vi "Begin.vi"(8 "error in":errorcluster) -> (0 "error out":errorcluster)   [LabVIEW 2018]
doc: "Called before other user functions, this VI is expected to open initial I/O refnums, load in file data, and do all program initialization. Notice that the <B>error out</B> terminal is simply used for data flow. Wiring it to other structures or subVIs ensures that this VI runs first."
uses:
  Robot Global Data.vi
  <vilib>/Rock Robotics/WPI/DriverStation/WPI_DriverStationRobotMode2.ctl
  <vilib>/Rock Robotics/WPI/Counter/WPI_CounterDigitalInputToDigitalSource.vi
  <vilib>/Rock Robotics/SystemInterfaces/DIO/FPGA_DIOChannel.ctl
  <vilib>/Rock Robotics/WPI/Solenoid/WPI_SolenoidOpenDouble.vi
  <vilib>/Rock Robotics/WPI/Solenoid/WPI_SolenoidSetEnum.vi
  <vilib>/Rock Robotics/WPI/Solenoid/WPI_SolenoidChannel.ctl
  <vilib>/Rock Robotics/SystemInterfaces/spilib/spi_bus.ctl
  <vilib>/Rock Robotics/WPI/Joystick/WPI_JoystickDeviceEnum.ctl
  <vilib>/Rock Robotics/SystemInterfaces/AI/FPGA_AIChannel.ctl
  <vilib>/Rock Robotics/WPI/Gyro/WPI_GyroXRS450_SPI_Open.vi
  <vilib>/Rock Robotics/WPI/Switch/WPI_SwitchOpenLimit.vi
  <vilib>/Rock Robotics/SystemInterfaces/DIO/FPGA_DIOPWMChannel.ctl
  <vilib>/Rock Robotics/WPI/PWM/WPI_PWMDeadband.ctl
  <vilib>/Rock Robotics/WPI/MotorControl/WPI_MotorControlType.ctl
  <vilib>/Rock Robotics/WPI/MotorControl/WPI_MotorControlDeviceRef.ctl
  <vilib>/Rock Robotics/WPI/RobotDrive/WPI_RobotDriveDevRef.ctl
  TeleopAutoCluster.ctl
  <vilib>/Rock Robotics/WPI/Joystick/WPI_JoystickDevRef.ctl
  <vilib>/Rock Robotics/WPI/Encoder/WPI_EncoderDevRef.ctl
  <vilib>/Rock Robotics/SystemInterfaces/Encoder/FPGA_EncoderIdx.ctl
  <vilib>/Rock Robotics/WPI/Encoder/WPI_EncoderType.ctl
  <vilib>/Rock Robotics/SystemInterfaces/Counter/FPGA_CounterCtrSystemIndex.ctl
  <vilib>/Rock Robotics/WPI/Gyro/WPI_GyroDevRef.ctl
  PTCluster.ctl
  <vilib>/Rock Robotics/WPI/Solenoid/WPI_SolenoidDevRef.ctl
  <vilib>/Rock Robotics/WPI/Switch/WPI_SwitchDevRef.ctl
  <vilib>/Rock Robotics/WPI/Potentiometer/WPI_PotentiometerDevRef.ctl
panel:
  out "PT Cluster Out":T1={"Elevator Encoder"={"DevStatus"={"status"=FALSE, "code"=0, "source"=""}, "EncoderIndex"=enum."Invalid", "CounterIndex"=enum."Ctr 1", "DistancePerCount"=2.0, "Decoding Type"=enum."4x"}, "Solenoid0"={"DevStatus"={"status"=FALSE, "code"=0, "source"=""}, "Pneumatics Control Module"=0, "Forward Solenoid Channel"=enum."Invalid", "Reverse Solenoid Channel"=enum."Invalid"}, "Solenoid1"={"DevStatus"={"status"=FALSE, "code"=0, "source"=""}, "Pneumatics Control Module"=0, "Forward Solenoid Channel"=enum."Invalid", "Reverse Solenoid Channel"=enum."Invalid"}, "Solenoid2"={"DevStatus"={"status"=FALSE, "code"=0, "source"=""}, "Pneumatics Control Module"=0, "Forward Solenoid Channel"=enum."Invalid", "Reverse Solenoid Channel"=enum."Invalid"}, "Solenoid3"={"DevStatus"={"status"=FALSE, "code"=0, "source"=""}, "Pneumatics Control Module"=0, "Forward Solenoid Channel"=enum."Invalid", "Reverse Solenoid Channel"=enum."Invalid"}, "Solenoid4"={"DevStatus"={"status"=FALSE, "code"=0, "source"=""}, "Pneumatics Control Module"=0, "Forward Solenoid Channel"=enum."Invalid", "Reverse Solenoid Channel"=enum."Invalid"}, "Elevator Master"={"DeviceStatus"={"status"=FALSE, "code"=0, "source"=""}, "Type"=enum."PWM", "PWM"={"PWM Channel"=enum."Invalid", "DeadBand"={"Name"="", "maxPositivePwm"=0, "minPositivePwm"=0, "centerPwm"=0, "maxNegativePwm"=0, "minNegativePwm"=0, "angularRange"=0}}, "CAN"={"Device Number"=0, "SetOutput VI Ref"=variant(refnum<vi> refnum), "GetOutput VI Ref"=variant(refnum<vi> refnum), "Enable VI Ref"=variant(refnum<vi> refnum), "Disable VI Ref"=variant(refnum<vi> refnum), "Data"=variant}, "Invert"=FALSE, "DIO PWM"={"PWM \"Enable\" Channel"=enum."Invalid", "DIOChannel"=enum."Invalid", "PWM Rate"=0.0}}, "Elevator Master 2"={"DeviceStatus"={"status"=FALSE, "code"=0, "source"=""}, "Type"=enum."PWM", "PWM"={"PWM Channel"=enum."Invalid", "DeadBand"={"Name"="", "maxPositivePwm"=0, "minPositivePwm"=0, "centerPwm"=0, "maxNegativePwm"=0, "minNegativePwm"=0, "angularRange"=0}}, "CAN"={"Device Number"=0, "SetOutput VI Ref"=variant(refnum<vi> refnum), "GetOutput VI Ref"=variant(refnum<vi> refnum), "Enable VI Ref"=variant(refnum<vi> refnum), "Disable VI Ref"=variant(refnum<vi> refnum), "Data"=variant}, "Invert"=FALSE, "DIO PWM"={"PWM \"Enable\" Channel"=enum."Invalid", "DIOChannel"=enum."Invalid", "PWM Rate"=0.0}}, "Elevator Master 3"={"DeviceStatus"={"status"=FALSE, "code"=0, "source"=""}, "Type"=enum."PWM", "PWM"={"PWM Channel"=enum."Invalid", "DeadBand"={"Name"="", "maxPositivePwm"=0, "minPositivePwm"=0, "centerPwm"=0, "maxNegativePwm"=0, "minNegativePwm"=0, "angularRange"=0}}, "CAN"={"Device Number"=0, "SetOutput VI Ref"=variant(refnum<vi> refnum), "GetOutput VI Ref"=variant(refnum<vi> refnum), "Enable VI Ref"=variant(refnum<vi> refnum), "Disable VI Ref"=variant(refnum<vi> refnum), "Data"=variant}, "Invert"=FALSE, "DIO PWM"={"PWM \"Enable\" Channel"=enum."Invalid", "DIOChannel"=enum."Invalid", "PWM Rate"=0.0}}, "Elevator Master 4"={"DeviceStatus"={"status"=FALSE, "code"=0, "source"=""}, "Type"=enum."PWM", "PWM"={"PWM Channel"=enum."Invalid", "DeadBand"={"Name"="", "maxPositivePwm"=0, "minPositivePwm"=0, "centerPwm"=0, "maxNegativePwm"=0, "minNegativePwm"=0, "angularRange"=0}}, "CAN"={"Device Number"=0, "SetOutput VI Ref"=variant(refnum<vi> refnum), "GetOutput VI Ref"=variant(refnum<vi> refnum), "Enable VI Ref"=variant(refnum<vi> refnum), "Disable VI Ref"=variant(refnum<vi> refnum), "Data"=variant}, "Invert"=FALSE, "DIO PWM"={"PWM \"Enable\" Channel"=enum."Invalid", "DIOChannel"=enum."Invalid", "PWM Rate"=0.0}}, "Elevator Bottom Out"={"DevStatus"={"status"=FALSE, "code"=0, "source"=""}, "DIO Channel"=enum."Invalid", "CntIndex"=enum."Invalid", "Normally Closed"=FALSE}, "Pot Moto"={"DevStatus"={"status"=FALSE, "code"=0, "source"=""}, "Analog Channel"=enum."Invalid", "Invert Output"=FALSE}, "Pot  Arm"={"DevStatus"={"status"=FALSE, "code"=0, "source"=""}, "Analog Channel"=enum."Invalid", "Invert Output"=FALSE}, "Elevator Master 5"={"DeviceStatus"={"status"=FALSE, "code"=0, "source"=""}, "Type"=enum."PWM", "PWM"={"PWM Channel"=enum."Invalid", "DeadBand"={"Name"="", "maxPositivePwm"=0, "minPositivePwm"=0, "centerPwm"=0, "maxNegativePwm"=0, "minNegativePwm"=0, "angularRange"=0}}, "CAN"={"Device Number"=0, "SetOutput VI Ref"=variant(refnum<vi> refnum), "GetOutput VI Ref"=variant(refnum<vi> refnum), "Enable VI Ref"=variant(refnum<vi> refnum), "Disable VI Ref"=variant(refnum<vi> refnum), "Data"=variant}, "Invert"=FALSE, "DIO PWM"={"PWM \"Enable\" Channel"=enum."Invalid", "DIOChannel"=enum."Invalid", "PWM Rate"=0.0}}, "Hatch Detection"={"DevStatus"={"status"=FALSE, "code"=0, "source"=""}, "DIO Channel"=enum."Invalid", "CntIndex"=enum."Invalid", "Normally Closed"=FALSE}, "Infrared"={"DevStatus"={"status"=FALSE, "code"=0, "source"=""}, "DIO Channel"=enum."Invalid", "CntIndex"=enum."Invalid", "Normally Closed"=FALSE}}
  in  "PT Cluster":T1={"Elevator Encoder"={"DevStatus"={"status"=FALSE, "code"=0, "source"=""}, "EncoderIndex"=enum."Invalid", "CounterIndex"=enum."Ctr 1", "DistancePerCount"=2.0, "Decoding Type"=enum."4x"}, "Solenoid0"={"DevStatus"={"status"=FALSE, "code"=0, "source"=""}, "Pneumatics Control Module"=0, "Forward Solenoid Channel"=enum."Invalid", "Reverse Solenoid Channel"=enum."Invalid"}, "Solenoid1"={"DevStatus"={"status"=FALSE, "code"=0, "source"=""}, "Pneumatics Control Module"=0, "Forward Solenoid Channel"=enum."Invalid", "Reverse Solenoid Channel"=enum."Invalid"}, "Solenoid2"={"DevStatus"={"status"=FALSE, "code"=0, "source"=""}, "Pneumatics Control Module"=0, "Forward Solenoid Channel"=enum."Invalid", "Reverse Solenoid Channel"=enum."Invalid"}, "Solenoid3"={"DevStatus"={"status"=FALSE, "code"=0, "source"=""}, "Pneumatics Control Module"=0, "Forward Solenoid Channel"=enum."Invalid", "Reverse Solenoid Channel"=enum."Invalid"}, "Solenoid4"={"DevStatus"={"status"=FALSE, "code"=0, "source"=""}, "Pneumatics Control Module"=0, "Forward Solenoid Channel"=enum."Invalid", "Reverse Solenoid Channel"=enum."Invalid"}, "Elevator Master"={"DeviceStatus"={"status"=FALSE, "code"=0, "source"=""}, "Type"=enum."PWM", "PWM"={"PWM Channel"=enum."Invalid", "DeadBand"={"Name"="", "maxPositivePwm"=0, "minPositivePwm"=0, "centerPwm"=0, "maxNegativePwm"=0, "minNegativePwm"=0, "angularRange"=0}}, "CAN"={"Device Number"=0, "SetOutput VI Ref"=variant(refnum<vi> refnum), "GetOutput VI Ref"=variant(refnum<vi> refnum), "Enable VI Ref"=variant(refnum<vi> refnum), "Disable VI Ref"=variant(refnum<vi> refnum), "Data"=variant}, "Invert"=FALSE, "DIO PWM"={"PWM \"Enable\" Channel"=enum."Invalid", "DIOChannel"=enum."Invalid", "PWM Rate"=0.0}}, "Elevator Master 2"={"DeviceStatus"={"status"=FALSE, "code"=0, "source"=""}, "Type"=enum."PWM", "PWM"={"PWM Channel"=enum."Invalid", "DeadBand"={"Name"="", "maxPositivePwm"=0, "minPositivePwm"=0, "centerPwm"=0, "maxNegativePwm"=0, "minNegativePwm"=0, "angularRange"=0}}, "CAN"={"Device Number"=0, "SetOutput VI Ref"=variant(refnum<vi> refnum), "GetOutput VI Ref"=variant(refnum<vi> refnum), "Enable VI Ref"=variant(refnum<vi> refnum), "Disable VI Ref"=variant(refnum<vi> refnum), "Data"=variant}, "Invert"=FALSE, "DIO PWM"={"PWM \"Enable\" Channel"=enum."Invalid", "DIOChannel"=enum."Invalid", "PWM Rate"=0.0}}, "Elevator Master 3"={"DeviceStatus"={"status"=FALSE, "code"=0, "source"=""}, "Type"=enum."PWM", "PWM"={"PWM Channel"=enum."Invalid", "DeadBand"={"Name"="", "maxPositivePwm"=0, "minPositivePwm"=0, "centerPwm"=0, "maxNegativePwm"=0, "minNegativePwm"=0, "angularRange"=0}}, "CAN"={"Device Number"=0, "SetOutput VI Ref"=variant(refnum<vi> refnum), "GetOutput VI Ref"=variant(refnum<vi> refnum), "Enable VI Ref"=variant(refnum<vi> refnum), "Disable VI Ref"=variant(refnum<vi> refnum), "Data"=variant}, "Invert"=FALSE, "DIO PWM"={"PWM \"Enable\" Channel"=enum."Invalid", "DIOChannel"=enum."Invalid", "PWM Rate"=0.0}}, "Elevator Master 4"={"DeviceStatus"={"status"=FALSE, "code"=0, "source"=""}, "Type"=enum."PWM", "PWM"={"PWM Channel"=enum."Invalid", "DeadBand"={"Name"="", "maxPositivePwm"=0, "minPositivePwm"=0, "centerPwm"=0, "maxNegativePwm"=0, "minNegativePwm"=0, "angularRange"=0}}, "CAN"={"Device Number"=0, "SetOutput VI Ref"=variant(refnum<vi> refnum), "GetOutput VI Ref"=variant(refnum<vi> refnum), "Enable VI Ref"=variant(refnum<vi> refnum), "Disable VI Ref"=variant(refnum<vi> refnum), "Data"=variant}, "Invert"=FALSE, "DIO PWM"={"PWM \"Enable\" Channel"=enum."Invalid", "DIOChannel"=enum."Invalid", "PWM Rate"=0.0}}, "Elevator Bottom Out"={"DevStatus"={"status"=FALSE, "code"=0, "source"=""}, "DIO Channel"=enum."Invalid", "CntIndex"=enum."Invalid", "Normally Closed"=FALSE}, "Pot Moto"={"DevStatus"={"status"=FALSE, "code"=0, "source"=""}, "Analog Channel"=enum."Invalid", "Invert Output"=FALSE}, "Pot  Arm"={"DevStatus"={"status"=FALSE, "code"=0, "source"=""}, "Analog Channel"=enum."Invalid", "Invert Output"=FALSE}, "Elevator Master 5"={"DeviceStatus"={"status"=FALSE, "code"=0, "source"=""}, "Type"=enum."PWM", "PWM"={"PWM Channel"=enum."Invalid", "DeadBand"={"Name"="", "maxPositivePwm"=0, "minPositivePwm"=0, "centerPwm"=0, "maxNegativePwm"=0, "minNegativePwm"=0, "angularRange"=0}}, "CAN"={"Device Number"=0, "SetOutput VI Ref"=variant(refnum<vi> refnum), "GetOutput VI Ref"=variant(refnum<vi> refnum), "Enable VI Ref"=variant(refnum<vi> refnum), "Disable VI Ref"=variant(refnum<vi> refnum), "Data"=variant}, "Invert"=FALSE, "DIO PWM"={"PWM \"Enable\" Channel"=enum."Invalid", "DIOChannel"=enum."Invalid", "PWM Rate"=0.0}}, "Hatch Detection"={"DevStatus"={"status"=FALSE, "code"=0, "source"=""}, "DIO Channel"=enum."Invalid", "CntIndex"=enum."Invalid", "Normally Closed"=FALSE}, "Infrared"={"DevStatus"={"status"=FALSE, "code"=0, "source"=""}, "DIO Channel"=enum."Invalid", "CntIndex"=enum."Invalid", "Normally Closed"=FALSE}}
  out "Teleop/Auto output cluster out":T16={"X Joystick"={"Device"=enum."USB 0"}, "Y Joystick"={"Device"=enum."USB 0"}, "Controller"={"Device"=enum."USB 0"}, "Right Drive Encoder"={"DevStatus"={"status"=FALSE, "code"=0, "source"=""}, "EncoderIndex"=enum."Invalid", "CounterIndex"=enum."Ctr 1", "DistancePerCount"=2.0, "Decoding Type"=enum."4x"}, "Left Drive Encoder"={"DevStatus"={"status"=FALSE, "code"=0, "source"=""}, "EncoderIndex"=enum."Invalid", "CounterIndex"=enum."Ctr 1", "DistancePerCount"=2.0, "Decoding Type"=enum."4x"}, "Gyro"={"DevStatus"={"status"=FALSE, "code"=0, "source"=""}, "Analog Channel"=enum."AI 1", "Gain (VoltsPerDegree/Second)"=0.0, "Gyro Type"=enum."Analog", "Handle"=0, "SPI Bus"=enum."Invalid", "Device Found"=FALSE, "Sample Rate"=1.0, "Calibrate On Open"=FALSE, "Offset"=0.0}, "DriveMotors"={"DevStatus"={"status"=FALSE, "code"=0, "source"=""}, "Motors[]"=[], "Square Inputs"=FALSE, "Max Output"=1.0}} {"Gyro"."Sample Rate" min=0.25 max=100.0 step=0.25}
  in  "Teleop/Auto output cluster":T16={"X Joystick"={"Device"=enum."USB 0"}, "Y Joystick"={"Device"=enum."USB 0"}, "Controller"={"Device"=enum."USB 0"}, "Right Drive Encoder"={"DevStatus"={"status"=FALSE, "code"=0, "source"=""}, "EncoderIndex"=enum."Invalid", "CounterIndex"=enum."Ctr 1", "DistancePerCount"=2.0, "Decoding Type"=enum."4x"}, "Left Drive Encoder"={"DevStatus"={"status"=FALSE, "code"=0, "source"=""}, "EncoderIndex"=enum."Invalid", "CounterIndex"=enum."Ctr 1", "DistancePerCount"=2.0, "Decoding Type"=enum."4x"}, "Gyro"={"DevStatus"={"status"=FALSE, "code"=0, "source"=""}, "Analog Channel"=enum."AI 1", "Gain (VoltsPerDegree/Second)"=0.0, "Gyro Type"=enum."Analog", "Handle"=0, "SPI Bus"=enum."Invalid", "Device Found"=FALSE, "Sample Rate"=1.0, "Calibrate On Open"=FALSE, "Offset"=0.0}, "DriveMotors"={"DevStatus"={"status"=FALSE, "code"=0, "source"=""}, "Motors[]"=[], "Square Inputs"=FALSE, "Max Output"=1.0}} {"Gyro"."Sample Rate" min=0.25 max=100.0 step=0.25}
  in  "RobotDriveDevRef":T21={"DevStatus"={"status"=FALSE, "code"=0, "source"=""}, "Motors[]"=[], "Square Inputs"=FALSE, "Max Output"=1.0}
  in  "DevStatus":errorcluster
  # "Analog"
  # "XRS"
  # "Analog"
  # "XRS"
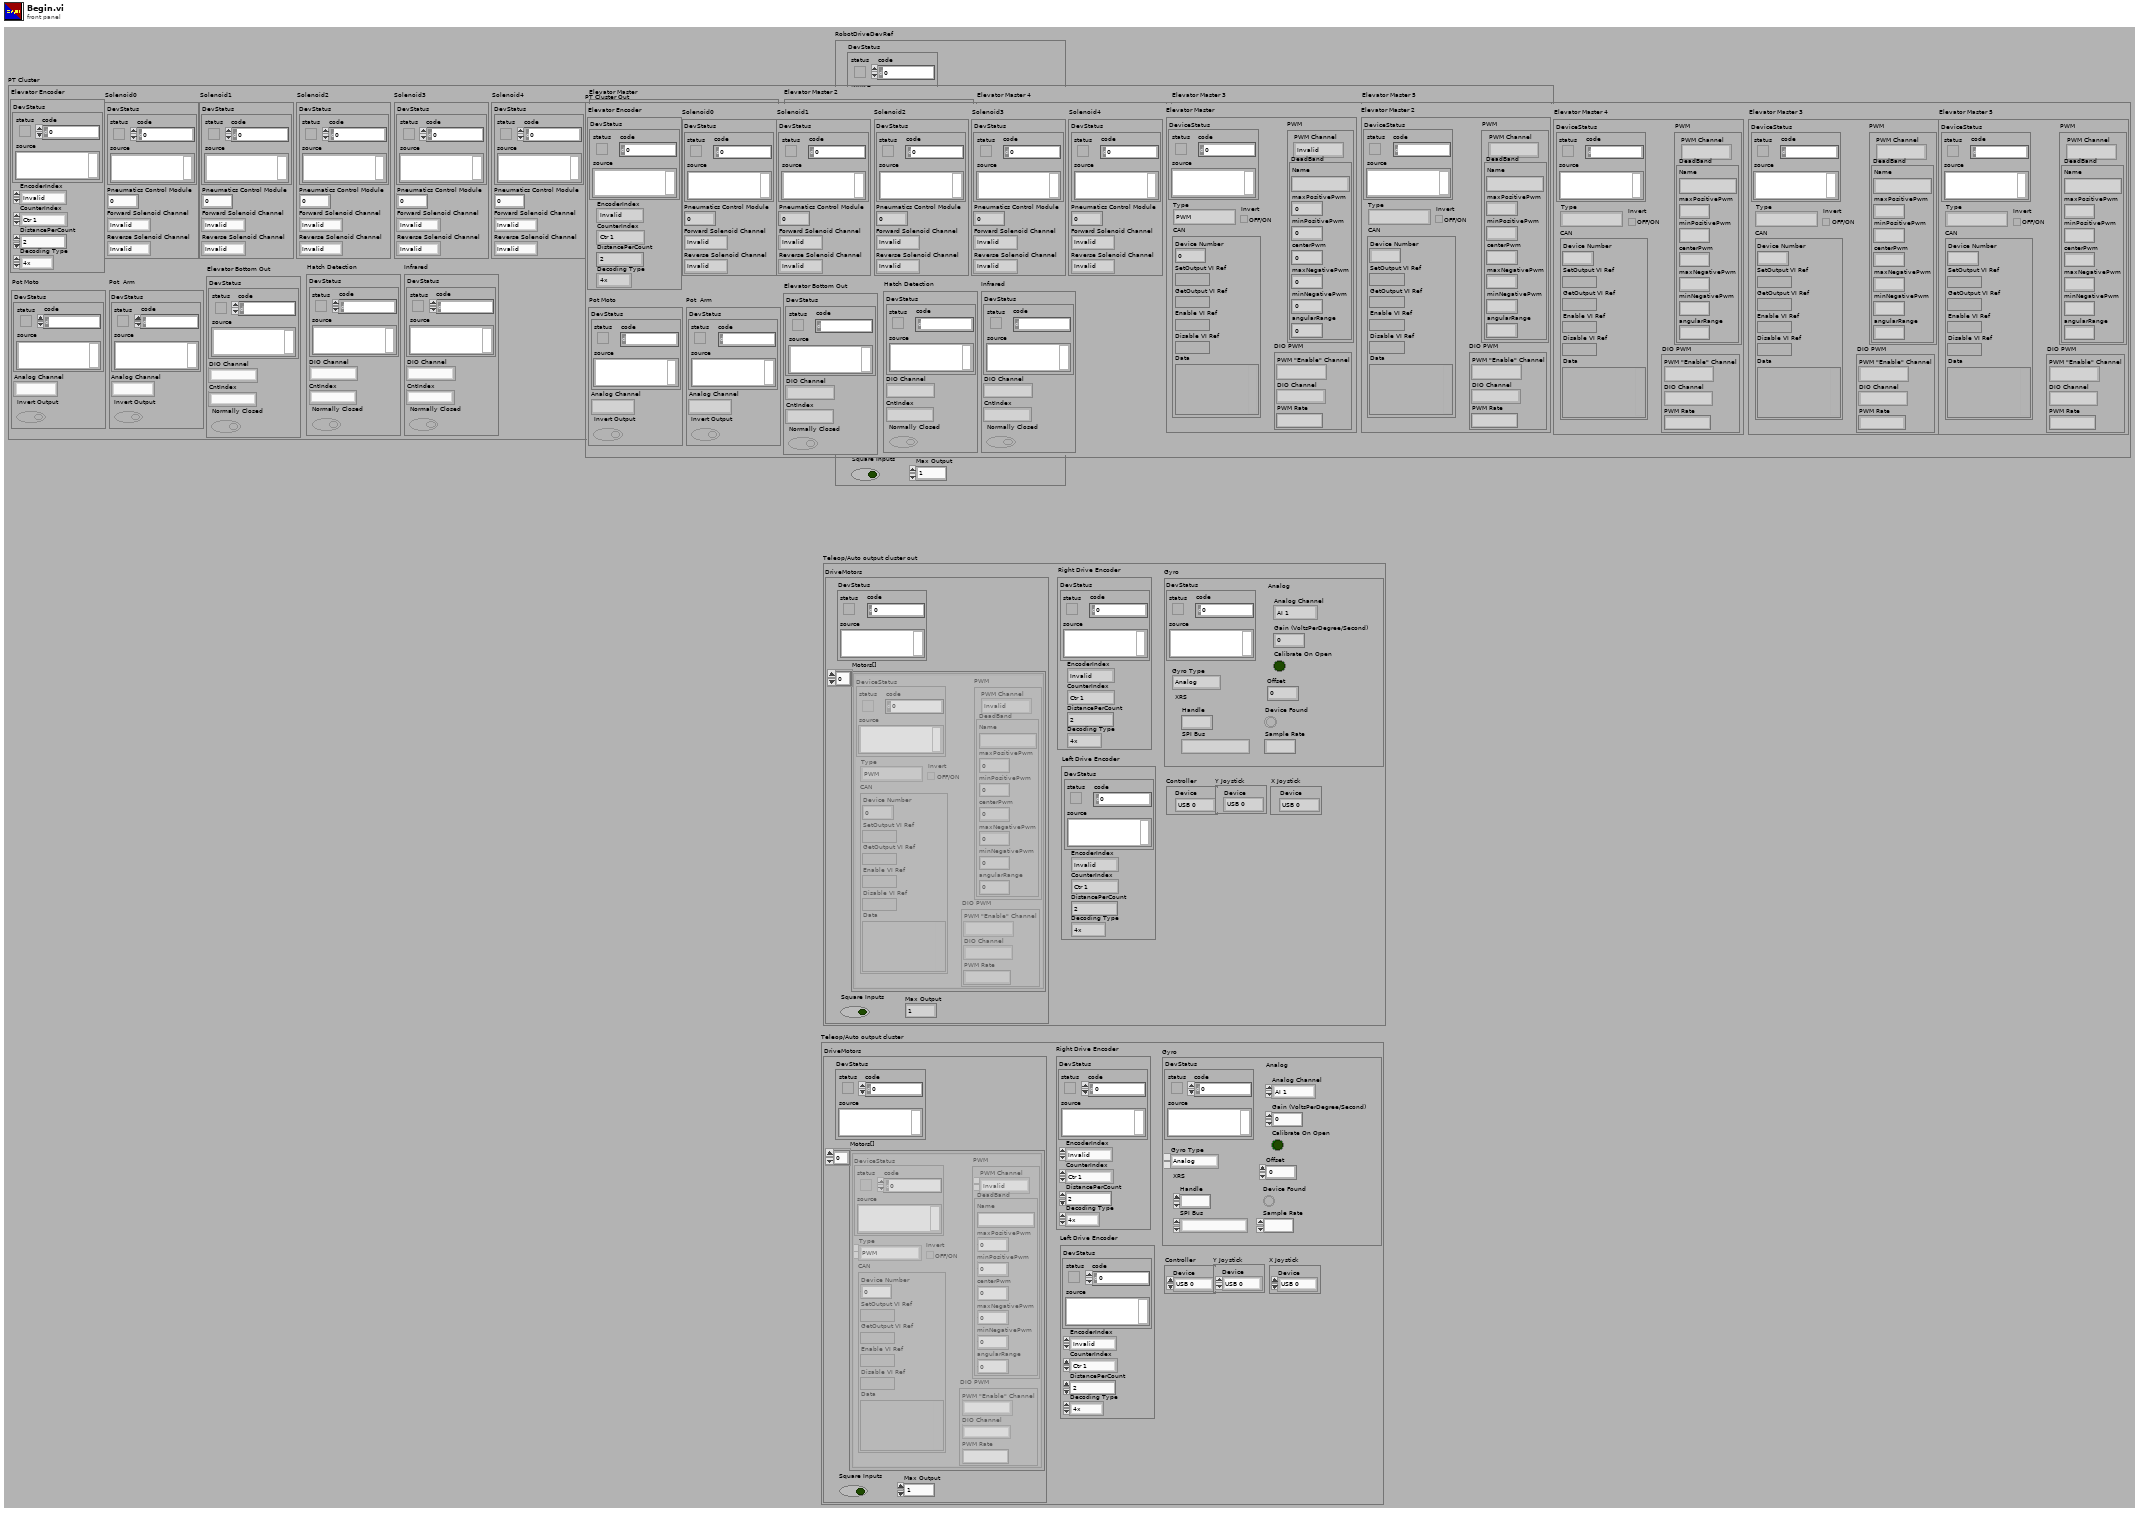
[diagram p1: front panel]
types:
  T1 = typedef "PTCluster.ctl" = cluster{"Elevator Encoder":T2, "Solenoid0":T6, "Solenoid1":T6, "Solenoid2":T6, "Solenoid3":T6, "Solenoid4":T6, "Elevator Master":T8, "Elevator Master 2":T8, "Elevator Master 3":T8, "Elevator Master 4":T8, "Elevator Bottom Out":T13, "Pot Moto":T14, "Pot  Arm":T14, "Elevator Master 5":T8, "Hatch Detection":T13, "Infrared":T13}
  T2 = typedef "WPI_EncoderDevRef.ctl" = cluster{"DevStatus":errorcluster, "EncoderIndex":T3, "CounterIndex":T4, "DistancePerCount":dbl, "Decoding Type":T5}
  T3 = typedef "FPGA_EncoderIdx.ctl" = enum8{"Enc 0", "Enc 1", "Enc 2", "Enc 3", "Enc 4", "Enc 5", "Enc 6", "Enc 7", "Invalid"}
  T4 = typedef "FPGA_CounterCtrSystemIndex.ctl" = enum8{"Ctr 0", "Ctr 1", "Ctr 2", "Ctr 3", "Ctr 4", "Ctr 5", "Ctr 6", "Ctr 7", "Invalid"}
  T5 = typedef "WPI_EncoderType.ctl" = enum16{"1x", "2x", "4x"}
  T6 = typedef "WPI_SolenoidDevRef.ctl" = cluster{"DevStatus":errorcluster, "Pneumatics Control Module":u8, "Forward Solenoid Channel":T7, "Reverse Solenoid Channel":T7}
  T7 = typedef "WPI_SolenoidChannel.ctl" = enum8{"Solenoid 0", "Solenoid 1", "Solenoid 2", "Solenoid 3", "Solenoid 4", "Solenoid 5", "Solenoid 6", "Solenoid 7", "Invalid"}
  T8 = typedef "WPI_MotorControlDeviceRef.ctl" = cluster{"DeviceStatus":errorcluster, "Type":T9, "PWM":cluster{"PWM Channel":T10, "DeadBand":T11}, "CAN":cluster{"Device Number":u8, "SetOutput VI Ref":variant, "GetOutput VI Ref":variant, "Enable VI Ref":variant, "Disable VI Ref":variant, "Data":variant}, "Invert":bool, "DIO PWM":cluster{"PWM \"Enable\" Channel":T10, "DIOChannel":T12, "PWM Rate":dbl}}
  T9 = typedef "WPI_MotorControlType.ctl" = enum16{"PWM", "CAN", "DIO PWM"}
  T10 = typedef "FPGA_DIOPWMChannel.ctl" = enum8{"PWM 0", "PWM 1", "PWM 2", "PWM 3", "PWM 4", "PWM 5", "PWM 6", "PWM 7", "PWM 8", "PWM 9", "PWM MXP 0", "PWM MXP 1", "PWM MXP 2", "PWM MXP 3", "PWM MXP 4", "PWM MXP 5", "PWM MXP 6", "PWM MXP 7", "PWM MXP 8", "PWM MXP 9", "Invalid"}
  T11 = typedef "WPI_PWMDeadband.ctl" = cluster{"Name":string, "maxPositivePwm":i32, "minPositivePwm":i32, "centerPwm":i32, "maxNegativePwm":i32, "minNegativePwm":i32, "angularRange":u16}
  T12 = typedef "FPGA_DIOChannel.ctl" = enum8{"DIO 0", "DIO 1", "DIO 2", "DIO 3", "DIO 4", "DIO 5", "DIO 6", "DIO 7", "DIO 8", "DIO 9", "DIO MXP 0", "DIO MXP 1", "DIO MXP 2", "DIO MXP 3", "DIO MXP 4", "DIO MXP 5", "DIO MXP 6", "DIO MXP 7", "DIO MXP 8", "DIO MXP 9", "DIO MXP 10", "DIO MXP 11", "DIO MXP 12", "DIO MXP 13", "DIO MXP 14", "DIO MXP 15", "SPI Port CS1", "SPI Port CS2", "SPI Port CS3", "SPI Port MISO", "SPI Port MOSI", "Invalid"}
  T13 = typedef "WPI_SwitchDevRef.ctl" = cluster{"DevStatus":errorcluster, "DIO Channel":T12, "CntIndex":T4, "Normally Closed":bool}
  T14 = typedef "WPI_PotentiometerDevRef.ctl" = cluster{"DevStatus":errorcluster, "Analog Channel":T15, "Invert Output":bool}
  T15 = typedef "FPGA_AIChannel.ctl" = enum8{"AI 0", "AI 1", "AI 2", "AI 3", "AI MXP 0", "AI MXP 1", "AI MXP 2", "AI MXP 3", "Invalid"}
  T16 = typedef "TeleopAutoCluster.ctl" = cluster{"X Joystick":T17, "Y Joystick":T17, "Controller":T17, "Right Drive Encoder":T2, "Left Drive Encoder":T2, "Gyro":T19, "DriveMotors":T21}
  T17 = typedef "WPI_JoystickDevRef.ctl" = cluster{"Device":T18}
  T18 = typedef "WPI_JoystickDeviceEnum.ctl" = enum16{"USB 0", "USB 1", "USB 2", "USB 3", "USB 4", "USB 5"}
  T19 = typedef "WPI_GyroDevRef.ctl" = cluster{"DevStatus":errorcluster, "Analog Channel":T15, "Gain (VoltsPerDegree/Second)":dbl, "Gyro Type":enum16{"Analog", "XRS450"}, "Handle":i32, "SPI Bus":T20, "Device Found":bool, "Sample Rate":dbl, "Calibrate On Open":bool, "Offset":dbl}
  T20 = typedef "spi_bus.ctl" = enum16{"SPI On-Board, CS0", "SPI On-Board, CS1", "SPI On-Board, CS2", "SPI On-Board, CS3", "SPI MXP", "Invalid"}
  T21 = typedef "WPI_RobotDriveDevRef.ctl" = cluster{"DevStatus":errorcluster, "Motors[]":T8[], "Square Inputs":bool, "Max Output":dbl}
  T22 = typedef "WPI_DriverStationRobotMode2.ctl" = enum16{"Autonomous Disabled", "Autonomous Enabled", "Teleop Disabled", "Teleop Enabled", "Disconnected", "Finish", "Test Disabled", "Test Enabled", "Emergency Stopped"}
  T23 = typedef "WPI_DigitalInputDevRef.ctl" = cluster{"DevStatus":errorcluster, "DIO Channel":T12}
  T24 = typedef "FPGA_CounterEncoderSourceConvertionLVSourceType.ctl" = cluster{"DevStatus":errorcluster, "AnalogTriggerMode?":bool, "DigitalMode":cluster{"DIO Channel":T25}, "AnalogTriggerMode":cluster{"AnalogTriggerIndex":T26, "OutputType":T27}}
  T25 = typedef "FPGA_DIODigitalSourceChannel.ctl" = enum8{"DIO 0", "DIO 1", "DIO 2", "DIO 3", "DIO 4", "DIO 5", "DIO 6", "DIO 7", "DIO 8", "DIO 9", "DIO MXP 0", "DIO MXP 1", "DIO MXP 2", "DIO MXP 3", "DIO MXP 4", "DIO MXP 5", "DIO MXP 6", "DIO MXP 7", "DIO MXP 8", "DIO MXP 9", "DIO MXP 10", "DIO MXP 11", "DIO MXP 12", "DIO MXP 13", "DIO MXP 14", "DIO MXP 15", "SPI Port CS1", "SPI Port CS2", "SPI Port CS3", "SPI Port MISO", "SPI Port MOSI", "Disabled"}
  T26 = typedef "FPGA_AnalogTriggerIndex.ctl" = enum8{"Trig 0", "Trig 1", "Trig 2", "Trig 3", "Trig 4", "Trig 5", "Trig 6", "Trig 7", "Invalid"}
  T27 = typedef "FPGA_AnalogTriggerOutType.ctl" = enum16{"InWindow", "TriggerState", "Rising", "Falling"}
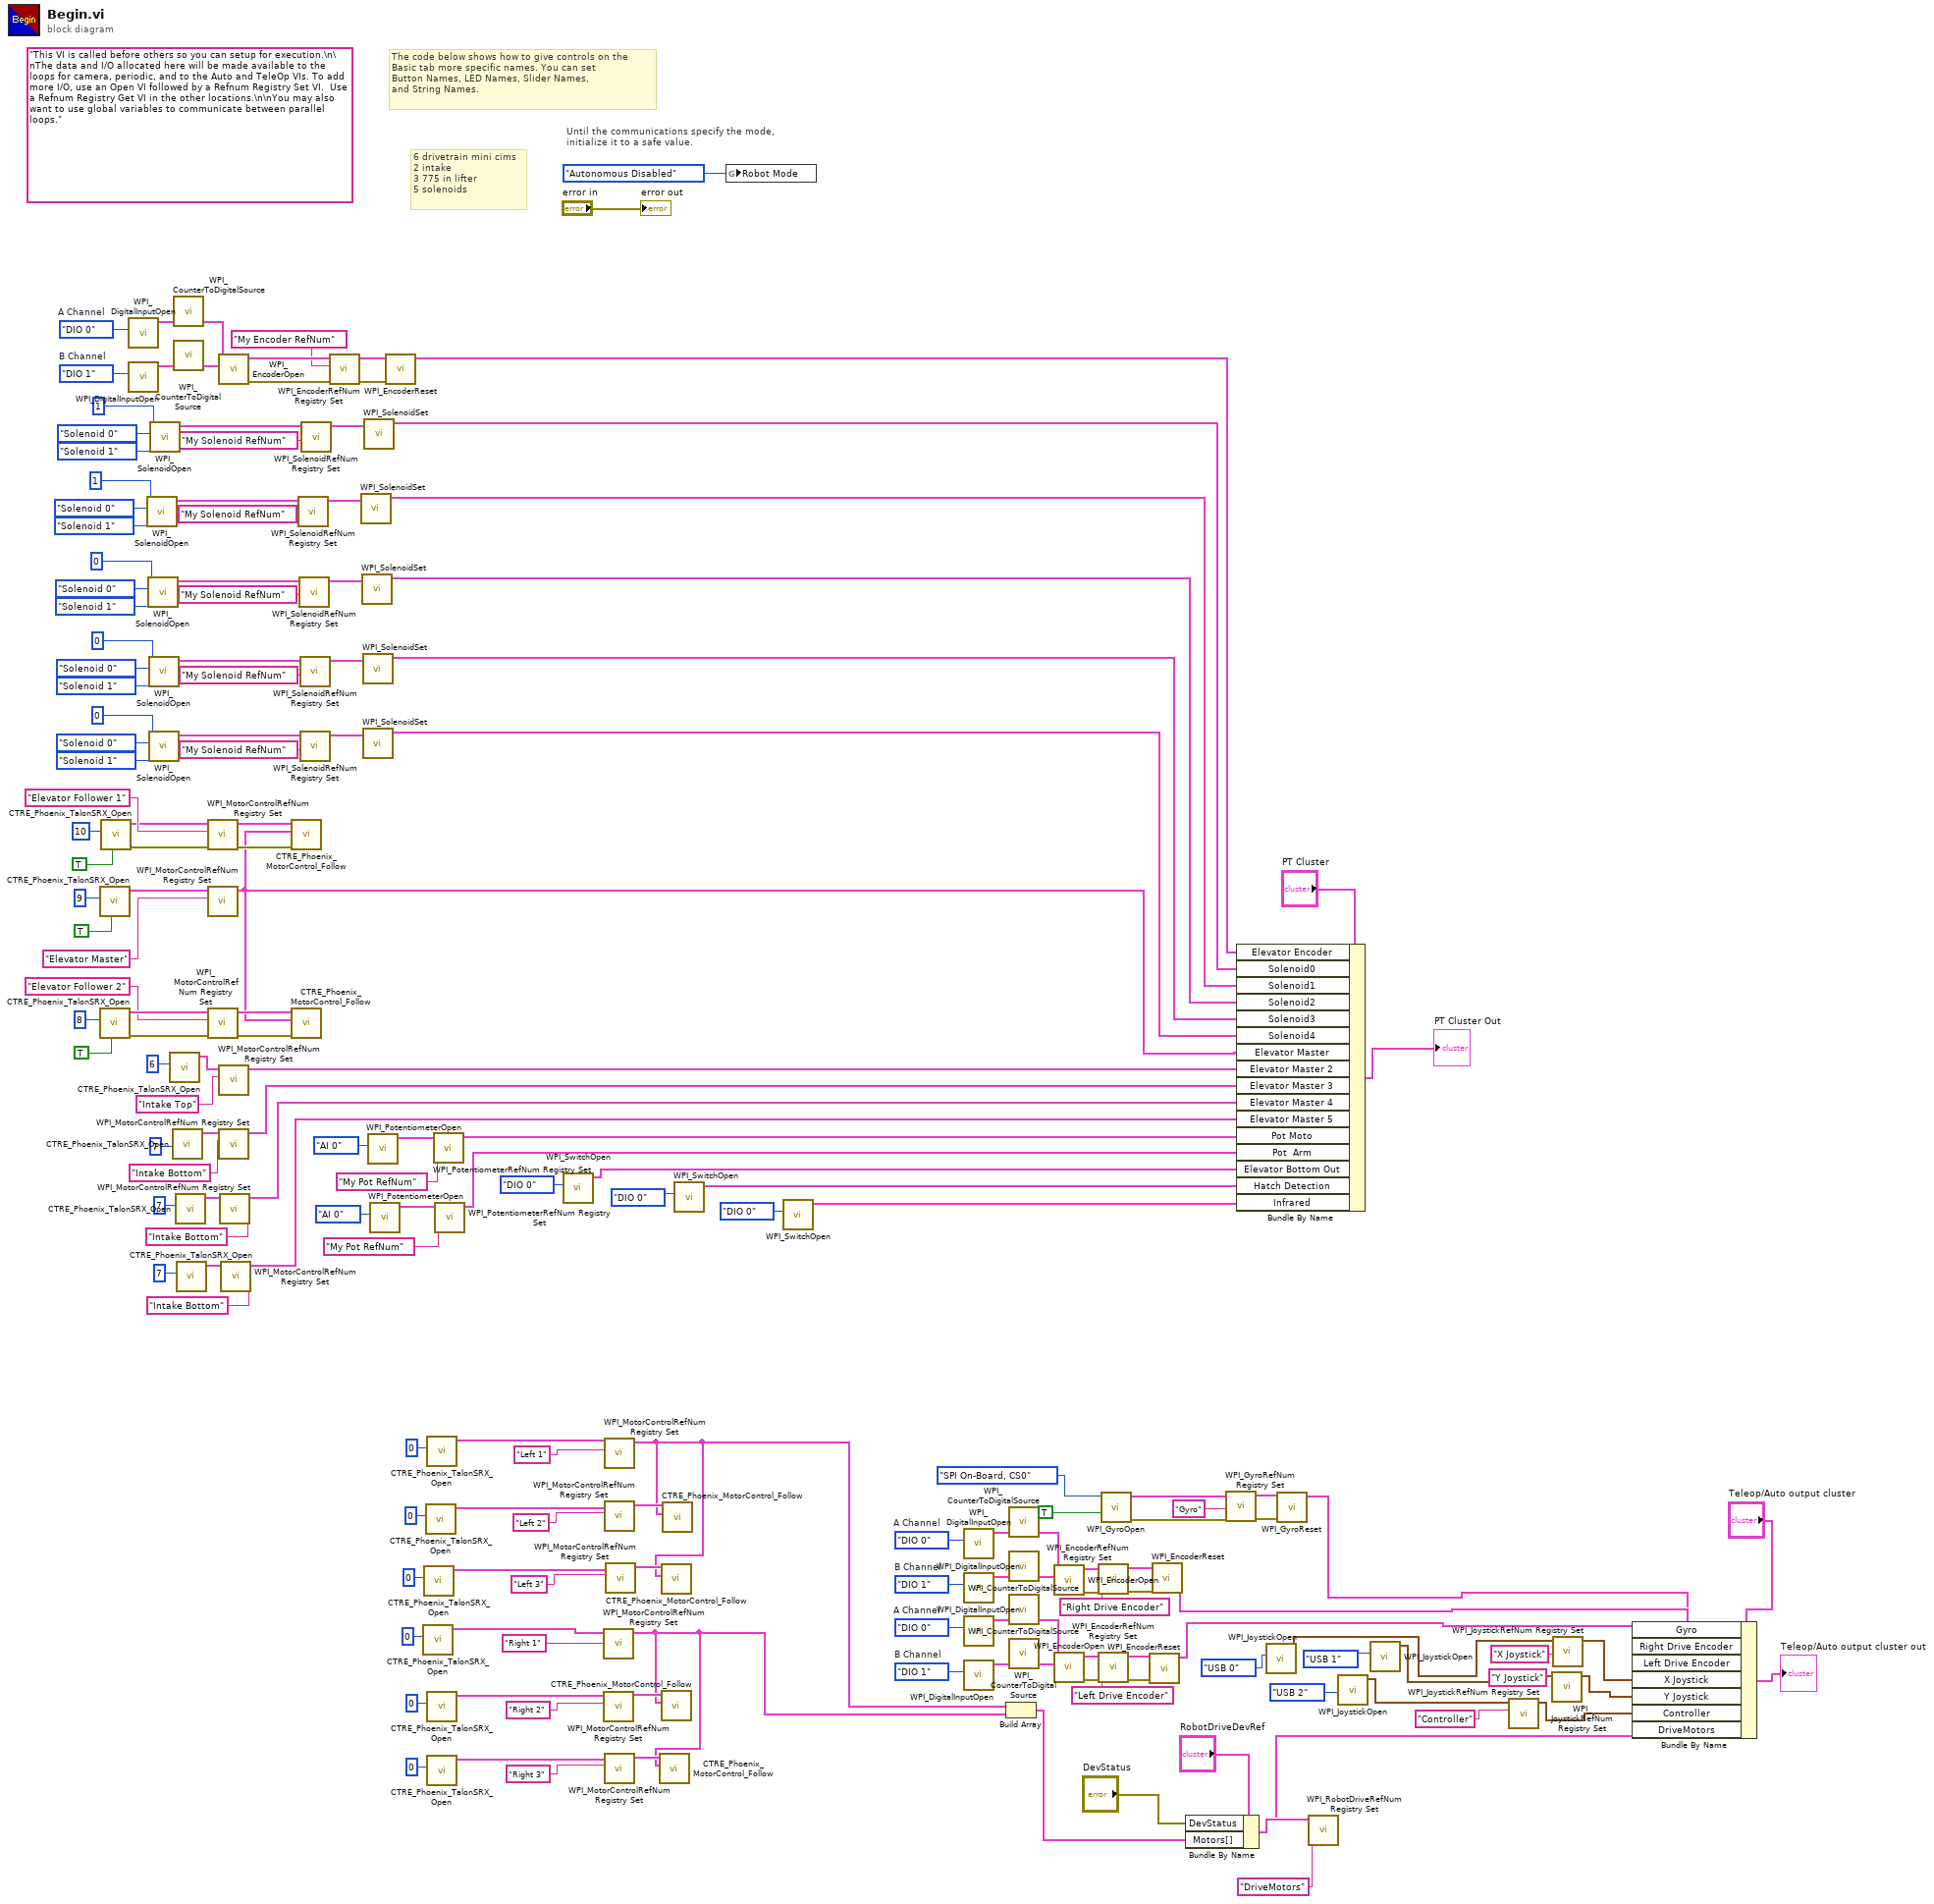
[diagram p0: block diagram]
diagram:
  w162 = FPGA_DIOChannel."DIO 1"  # B Channel
  w161 = FPGA_DIOChannel."DIO 0"  # A Channel
  w168 = FPGA_DIOChannel."DIO 1"  # B Channel
  w167 = FPGA_DIOChannel."DIO 0"  # A Channel
  w174 = FPGA_DIOChannel."DIO 1"  # B Channel
  w173 = FPGA_DIOChannel."DIO 0"  # A Channel
  (unwired) "This VI is called before others so you can setup for execution.\n\nThe data and I/O allocated here will be made available to the loops for camera, periodic, and to the Auto and TeleOp VIs. To add more I/O, use an Open VI followed by a Refnum Registry Set VI.  Use a Refnum Registry Get VI in the other locations.\n\nYou may also want to use global variables to communicate between parallel loops."
  # "6 drivetrain mini cims\n2 intake\n3 775 in lifter\n5 solenoids"
  # "The code below shows how to give controls on the\nBasic tab more specific names. You can set\nButton Names, LED Names, Slider Names,\nand String Names."
  # "Until the communications specify the mode,\ninitialize it to a safe value."
  n1 = call <vilib>:"CTRE_Phoenix_TalonSRX_Open.vi"("Invert"=TRUE, "Device Number"=u8 9) -> ("CAN Talon SRX Ref"=w111:T8)  [unwired: 8 in, 1 out]
  n2 = call <vilib>:"CTRE_Phoenix_TalonSRX_Open.vi"("Invert"=TRUE, "Device Number"=u8 8) -> ("error out"=w100:errorcluster, "CAN Talon SRX Ref"=w97:T8)  [unwired: 8 in]
  n3 = call <vilib>:"CTRE_Phoenix_TalonSRX_Open.vi"("Invert"=TRUE, "Device Number"=u8 10) -> ("error out"=w105:errorcluster, "CAN Talon SRX Ref"=w108:T8)  [unwired: 8 in]
  n4 = call <vilib>:"WPI_DigitalInputOpen.vi"("DIO Channel"=w173) -> ("DigitalInputDevRef"=w170:T23)  [unwired: 1 in, 9 out]
  n5 = call <vilib>:"WPI_DigitalInputOpen.vi"("DIO Channel"=w174) -> ("DigitalInputDevRef"=w171:T23)  [unwired: 1 in, 9 out]
  n6 = call-poly <vilib>:"WPI_SolenoidOpen.vi"("Reverse Solenoid Channel"=WPI_SolenoidChannel."Solenoid 1", "Forward Solenoid Channel"=WPI_SolenoidChannel."Solenoid 0", "Pneumatics Control Module (0)"=u8 1) -> ("SolenoidDevRef"=w114:T6)  [unwired: 7 in, 1 out]
  n7 = call-poly <vilib>:"WPI_SolenoidOpen.vi"("Reverse Solenoid Channel"=WPI_SolenoidChannel."Solenoid 1", "Forward Solenoid Channel"=WPI_SolenoidChannel."Solenoid 0", "Pneumatics Control Module (0)"=u8 0) -> ("SolenoidDevRef"=w128:T6)  [unwired: 7 in, 1 out]
  n8 = call-poly <vilib>:"WPI_SolenoidOpen.vi"("Reverse Solenoid Channel"=WPI_SolenoidChannel."Solenoid 1", "Forward Solenoid Channel"=WPI_SolenoidChannel."Solenoid 0", "Pneumatics Control Module (0)"=u8 0) -> ("SolenoidDevRef"=w129:T6)  [unwired: 7 in, 1 out]
  n9 = call-poly <vilib>:"WPI_SolenoidOpen.vi"("Reverse Solenoid Channel"=WPI_SolenoidChannel."Solenoid 1", "Forward Solenoid Channel"=WPI_SolenoidChannel."Solenoid 0", "Pneumatics Control Module (0)"=u8 0) -> ("SolenoidDevRef"=w144:T6)  [unwired: 7 in, 1 out]
  n10 = call-poly <vilib>:"WPI_SolenoidOpen.vi"("Reverse Solenoid Channel"=WPI_SolenoidChannel."Solenoid 1", "Forward Solenoid Channel"=WPI_SolenoidChannel."Solenoid 0", "Pneumatics Control Module (0)"=u8 1) -> ("SolenoidDevRef"=w123:T6)  [unwired: 7 in, 1 out]
  n11 = call <vilib>:"CTRE_Phoenix_TalonSRX_Open.vi"("Device Number"=u8 6) -> ("CAN Talon SRX Ref"=w61:T8)  [unwired: 9 in, 1 out]
  n12 = call <vilib>:"CTRE_Phoenix_TalonSRX_Open.vi"("Device Number"=u8 7) -> ("CAN Talon SRX Ref"=w53:T8)  [unwired: 9 in, 1 out]
  n13 = call-poly <vilib>:"WPI_CounterToDigitalSource.vi"("DigitalInputDevRef"=w170) -> ("Digital Source"=w169:T24)  [unwired: 6 out]
  n14 = call-poly <vilib>:"WPI_CounterToDigitalSource.vi"("DigitalInputDevRef"=w171) -> ("Digital Source"=w172:T24)  [unwired: 6 out]
  n15 = call <vilib>:"CTRE_Phoenix_TalonSRX_Open.vi"("Device Number"=u8 7) -> ("CAN Talon SRX Ref"=w56:T8)  [unwired: 9 in, 1 out]
  n16 = call <vilib>:"CTRE_Phoenix_TalonSRX_Open.vi"("Device Number"=u8 7) -> ("CAN Talon SRX Ref"=w59:T8)  [unwired: 9 in, 1 out]
  n17 = call <vilib>:"WPI_MotorControlRefNum Registry Set.vi"("error in (no error)"=w105, "refnum name"="Elevator Follower 1", "MotorControlDevRef"=w108) -> ("error out"=w104:errorcluster, "MotorControlDevRef"=w106:T8)  [unwired: 7 in]
  n18 = call <vilib>:"WPI_MotorControlRefNum Registry Set.vi"("refnum name"="Elevator Master", "MotorControlDevRef"=w111) -> ("MotorControlDevRef"=w12:T8)  [unwired: 8 in, 1 out]
  n19 = call <vilib>:"WPI_MotorControlRefNum Registry Set.vi"("error in (no error)"=w100, "refnum name"="Elevator Follower 2", "MotorControlDevRef"=w97) -> ("error out"=w101:errorcluster, "MotorControlDevRef"=w99:T8)  [unwired: 7 in]
  n20 = call <vilib>:"WPI_EncoderOpen.vi"("BSource"=w172, "ASource"=w169) -> ("error out"=w156:errorcluster, "EncoderDevRef"=w155:T2)  [unwired: 6 in, 2 out]
  n21 = call <vilib>:"WPI_MotorControlRefNum Registry Set.vi"("refnum name"="Intake Top", "MotorControlDevRef"=w61) -> ("MotorControlDevRef"=w11:T8)  [unwired: 8 in, 1 out]
  n22 = call <vilib>:"WPI_MotorControlRefNum Registry Set.vi"("refnum name"="Intake Bottom", "MotorControlDevRef"=w53) -> ("MotorControlDevRef"=w10:T8)  [unwired: 8 in, 1 out]
  n23 = call <vilib>:"WPI_MotorControlRefNum Registry Set.vi"("refnum name"="Intake Bottom", "MotorControlDevRef"=w56) -> ("MotorControlDevRef"=w9:T8)  [unwired: 8 in, 1 out]
  n24 = call <vilib>:"WPI_MotorControlRefNum Registry Set.vi"("refnum name"="Intake Bottom", "MotorControlDevRef"=w59) -> ("MotorControlDevRef"=w8:T8)  [unwired: 8 in, 1 out]
  n25 = call <vilib>:"CTRE_Phoenix_MotorControl_Follow.vi"("error in (no error)"=w104, "Master Controller to Follow"=w12, "PhoenixMotorControlDevRef"=w106) -> ()  [unwired: 7 in, 2 out]
  n26 = call <vilib>:"CTRE_Phoenix_MotorControl_Follow.vi"("error in (no error)"=w101, "Master Controller to Follow"=w12, "PhoenixMotorControlDevRef"=w99) -> ()  [unwired: 7 in, 2 out]
  n27 = call <vilib>:"WPI_SolenoidRefNum Registry Set.vi"("refnum name"="My Solenoid RefNum", "SolenoidDevRef"=w114) -> ("SolenoidDevRef"=w115:T6)  [unwired: 8 in, 1 out]
  n28 = call <vilib>:"WPI_SolenoidRefNum Registry Set.vi"("refnum name"="My Solenoid RefNum", "SolenoidDevRef"=w128) -> ("SolenoidDevRef"=w127:T6)  [unwired: 8 in, 1 out]
  n29 = call <vilib>:"WPI_SolenoidRefNum Registry Set.vi"("refnum name"="My Solenoid RefNum", "SolenoidDevRef"=w129) -> ("SolenoidDevRef"=w130:T6)  [unwired: 8 in, 1 out]
  n30 = call <vilib>:"WPI_SolenoidRefNum Registry Set.vi"("refnum name"="My Solenoid RefNum", "SolenoidDevRef"=w144) -> ("SolenoidDevRef"=w143:T6)  [unwired: 8 in, 1 out]
  n31 = call <vilib>:"WPI_SolenoidRefNum Registry Set.vi"("refnum name"="My Solenoid RefNum", "SolenoidDevRef"=w123) -> ("SolenoidDevRef"=w122:T6)  [unwired: 8 in, 1 out]
  n32 = call <vilib>:"WPI_EncoderRefNum Registry Set.vi"("error in (no error)"=w156, "refnum name"="My Encoder RefNum", "EncoderDevRef"=w155) -> ("error out"=w154:errorcluster, "EncoderDevRef"=w153:T2)  [unwired: 7 in]
  n33 = call-poly <vilib>:"WPI_SolenoidSet.vi"("SolenoidDevRef"=w115) -> ("SolenoidDevRef"=w16:T6)  [unwired: 9 in, 1 out]
  n34 = call-poly <vilib>:"WPI_SolenoidSet.vi"("SolenoidDevRef"=w127) -> ("SolenoidDevRef"=w15:T6)  [unwired: 9 in, 1 out]
  n35 = call-poly <vilib>:"WPI_SolenoidSet.vi"("SolenoidDevRef"=w130) -> ("SolenoidDevRef"=w14:T6)  [unwired: 9 in, 1 out]
  n36 = call-poly <vilib>:"WPI_SolenoidSet.vi"("SolenoidDevRef"=w143) -> ("SolenoidDevRef"=w13:T6)  [unwired: 9 in, 1 out]
  n37 = call-poly <vilib>:"WPI_SolenoidSet.vi"("SolenoidDevRef"=w122) -> ("SolenoidDevRef"=w17:T6)  [unwired: 9 in, 1 out]
  n38 = call <vilib>:"WPI_PotentiometerOpen.vi"("Analog Channel"=FPGA_AIChannel."AI 0") -> ("PotDevRef"=w48:T14)  [unwired: 9 in, 1 out]
  n39 = call <vilib>:"WPI_PotentiometerOpen.vi"("Analog Channel"=FPGA_AIChannel."AI 0") -> ("PotDevRef"=w49:T14)  [unwired: 9 in, 1 out]
  n40 = call <vilib>:"WPI_EncoderReset.vi"("error in (no error)"=w154, "EncoderDevRef"=w153) -> ("EncoderDevRef"=w18:T2)  [unwired: 8 in, 1 out]
  n41 = call <vilib>:"CTRE_Phoenix_TalonSRX_Open.vi"("Device Number"=u8 0) -> ("CAN Talon SRX Ref"=w81:T8)  [unwired: 9 in, 1 out]
  n42 = call <vilib>:"CTRE_Phoenix_TalonSRX_Open.vi"("Device Number"=u8 0) -> ("CAN Talon SRX Ref"=w80:T8)  [unwired: 9 in, 1 out]
  n43 = call <vilib>:"CTRE_Phoenix_TalonSRX_Open.vi"("Device Number"=u8 0) -> ("CAN Talon SRX Ref"=w79:T8)  [unwired: 9 in, 1 out]
  n44 = call <vilib>:"CTRE_Phoenix_TalonSRX_Open.vi"("Device Number"=u8 0) -> ("CAN Talon SRX Ref"=w78:T8)  [unwired: 9 in, 1 out]
  n45 = call <vilib>:"CTRE_Phoenix_TalonSRX_Open.vi"("Device Number"=u8 0) -> ("CAN Talon SRX Ref"=w82:T8)  [unwired: 9 in, 1 out]
  n46 = call <vilib>:"CTRE_Phoenix_TalonSRX_Open.vi"("Device Number"=u8 0) -> ("CAN Talon SRX Ref"=w83:T8)  [unwired: 9 in, 1 out]
  n47 = call <vilib>:"WPI_PotentiometerRefNum Registry Set.vi"("refnum name"="My Pot RefNum", "PotDevRef"=w48) -> ("PotDevRef"=w7:T14)  [unwired: 8 in, 1 out]
  n48 = call <vilib>:"WPI_PotentiometerRefNum Registry Set.vi"("refnum name"="My Pot RefNum", "PotDevRef"=w49) -> ("PotDevRef"=w6:T14)  [unwired: 8 in, 1 out]
  n49 = call-poly <vilib>:"WPI_SwitchOpen.vi"("DIO Channel"=FPGA_DIOChannel."DIO 0") -> ("SwitchDevRef"=w5:T13)  [unwired: 9 in, 1 out]
  n50 = call <vilib>:"WPI_MotorControlRefNum Registry Set.vi"("refnum name"="Right 1", "MotorControlDevRef"=w81) -> ("MotorControlDevRef"=w41:T8)  [unwired: 8 in, 1 out]
  n51 = call <vilib>:"WPI_MotorControlRefNum Registry Set.vi"("refnum name"="Right 2", "MotorControlDevRef"=w82) -> ("MotorControlDevRef"=w43:T8)  [unwired: 8 in, 1 out]
  n52 = call <vilib>:"WPI_MotorControlRefNum Registry Set.vi"("refnum name"="Left 1", "MotorControlDevRef"=w78) -> ("MotorControlDevRef"=w44:T8)  [unwired: 8 in, 1 out]
  n53 = call <vilib>:"WPI_MotorControlRefNum Registry Set.vi"("refnum name"="Left 2", "MotorControlDevRef"=w79) -> ("MotorControlDevRef"=w46:T8)  [unwired: 8 in, 1 out]
  n54 = call <vilib>:"WPI_MotorControlRefNum Registry Set.vi"("refnum name"="Right 3", "MotorControlDevRef"=w83) -> ("MotorControlDevRef"=w42:T8)  [unwired: 8 in, 1 out]
  n55 = call <vilib>:"WPI_MotorControlRefNum Registry Set.vi"("refnum name"="Left 3", "MotorControlDevRef"=w80) -> ("MotorControlDevRef"=w45:T8)  [unwired: 8 in, 1 out]
  n56 = call <vilib>:"CTRE_Phoenix_MotorControl_Follow.vi"("Master Controller to Follow"=w41, "PhoenixMotorControlDevRef"=w42) -> ()  [unwired: 8 in, 2 out]
  n57 = call <vilib>:"CTRE_Phoenix_MotorControl_Follow.vi"("Master Controller to Follow"=w44, "PhoenixMotorControlDevRef"=w45) -> ()  [unwired: 8 in, 2 out]
  n58 = call <vilib>:"CTRE_Phoenix_MotorControl_Follow.vi"("Master Controller to Follow"=w41, "PhoenixMotorControlDevRef"=w43) -> ()  [unwired: 8 in, 2 out]
  n59 = call <vilib>:"CTRE_Phoenix_MotorControl_Follow.vi"("Master Controller to Follow"=w44, "PhoenixMotorControlDevRef"=w46) -> ()  [unwired: 8 in, 2 out]
  n60 = call-poly <vilib>:"WPI_SwitchOpen.vi"("DIO Channel"=FPGA_DIOChannel."DIO 0") -> ("SwitchDevRef"=w2:T13)  [unwired: 9 in, 1 out]
  n61 = global write "Robot Global Data.vi" "Robot Mode"(WPI_DriverStationRobotMode2."Autonomous Disabled" ("Robot Mode")) -> ()
  n62 = call-poly <vilib>:"WPI_SwitchOpen.vi"("DIO Channel"=FPGA_DIOChannel."DIO 0") -> ("SwitchDevRef"=w1:T13)  [unwired: 9 in, 1 out]
  n63 = call <vilib>:"WPI_DigitalInputOpen.vi"("DIO Channel"=w167) -> ("DigitalInputDevRef"=w164:T23)  [unwired: 1 in, 9 out]
  n64 = call <vilib>:"WPI_DigitalInputOpen.vi"("DIO Channel"=w168) -> ("DigitalInputDevRef"=w165:T23)  [unwired: 1 in, 9 out]
  n65 = call <vilib>:"WPI_DigitalInputOpen.vi"("DIO Channel"=w161) -> ("DigitalInputDevRef"=w158:T23)  [unwired: 1 in, 9 out]
  n66 = call <vilib>:"WPI_DigitalInputOpen.vi"("DIO Channel"=w162) -> ("DigitalInputDevRef"=w159:T23)  [unwired: 1 in, 9 out]
  n67 = Build Array(w44, w41) -> (w40:T8[])
  n68 = call-poly <vilib>:"WPI_CounterToDigitalSource.vi"("DigitalInputDevRef"=w164) -> ("Digital Source"=w163:T24)  [unwired: 6 out]
  n69 = call-poly <vilib>:"WPI_CounterToDigitalSource.vi"("DigitalInputDevRef"=w165) -> ("Digital Source"=w166:T24)  [unwired: 6 out]
  n70 = call-poly <vilib>:"WPI_CounterToDigitalSource.vi"("DigitalInputDevRef"=w158) -> ("Digital Source"=w157:T24)  [unwired: 6 out]
  n71 = call-poly <vilib>:"WPI_CounterToDigitalSource.vi"("DigitalInputDevRef"=w159) -> ("Digital Source"=w160:T24)  [unwired: 6 out]
  n72 = call <vilib>:"WPI_EncoderOpen.vi"("BSource"=w166, "ASource"=w163) -> ("error out"=w152:errorcluster, "EncoderDevRef"=w151:T2)  [unwired: 6 in, 2 out]
  n73 = call <vilib>:"WPI_EncoderOpen.vi"("BSource"=w160, "ASource"=w157) -> ("error out"=w148:errorcluster, "EncoderDevRef"=w147:T2)  [unwired: 6 in, 2 out]
  n74 = call <vilib>:"WPI_EncoderRefNum Registry Set.vi"("error in (no error)"=w152, "refnum name"="Right Drive Encoder", "EncoderDevRef"=w151) -> ("error out"=w150:errorcluster, "EncoderDevRef"=w149:T2)  [unwired: 7 in]
  n75 = call <vilib>:"WPI_EncoderRefNum Registry Set.vi"("error in (no error)"=w148, "refnum name"="Left Drive Encoder", "EncoderDevRef"=w147) -> ("error out"=w146:errorcluster, "EncoderDevRef"=w145:T2)  [unwired: 7 in]
  n76 = call-poly <vilib>:"WPI_GyroOpen.vi"("Calibrate On Open"=TRUE, "SPI Bus"=spi_bus."SPI On-Board, CS0") -> ("error out"=w135:errorcluster, "GyroDevRef"=w137:T19)  [unwired: 7 in, 1 out]
  n77 = call <vilib>:"WPI_EncoderReset.vi"("error in (no error)"=w146, "EncoderDevRef"=w145) -> ("EncoderDevRef"=w65:T2)  [unwired: 8 in, 1 out]
  n78 = call <vilib>:"WPI_EncoderReset.vi"("error in (no error)"=w150, "EncoderDevRef"=w149) -> ("EncoderDevRef"=w64:T2)  [unwired: 8 in, 1 out]
  n79 = Bundle By Name(cluster="RobotDriveDevRef", "DevStatus"="DevStatus", "Motors[]"=w40) -> (w69:T21)
  n80 = call <vilib>:"WPI_GyroRefNum Registry Set.vi"("error in (no error)"=w135, "refnum name"="Gyro", "GyroDevRef"=w137) -> ("error out"=w139:errorcluster, "GyroDevRef"=w138:T19)  [unwired: 7 in]
  n81 = Bundle By Name(cluster="PT Cluster", "Elevator Encoder"=w18, "Solenoid0"=w17, "Solenoid1"=w16, "Solenoid2"=w15, "Solenoid3"=w14, "Solenoid4"=w13, "Elevator Master"=w12, "Elevator Master 2"=w11, "Elevator Master 3"=w10, "Elevator Master 4"=w9, "Elevator Master 5"=w8, "Pot Moto"=w7, "Pot  Arm"=w6, "Elevator Bottom Out"=w5, "Hatch Detection"=w2, "Infrared"=w1) -> (→"PT Cluster Out":T1)
  n82 = call <vilib>:"WPI_JoystickOpen.vi"("JoystickDevice"=WPI_JoystickDeviceEnum."USB 0") -> ("JoystickDevRef"=w27:T17)  [unwired: 10 in]
  n83 = call <vilib>:"WPI_GyroReset.vi"("error in"=w139, "GyroDevRef"=w138) -> ("GyroDevRef"=w63:T19)  [unwired: 8 in, 1 out]
  n84 = call <vilib>:"WPI_RobotDriveRefNum Registry Set.vi"("refnum name"="DriveMotors", "RobotDriveDevRef"=w69) -> ("RobotDriveDevRef"=w66:T21)  [unwired: 8 in, 1 out]
  n85 = call <vilib>:"WPI_JoystickOpen.vi"("JoystickDevice"=WPI_JoystickDeviceEnum."USB 2") -> ("JoystickDevRef"=w29:T17)  [unwired: 10 in]
  n86 = call <vilib>:"WPI_JoystickOpen.vi"("JoystickDevice"=WPI_JoystickDeviceEnum."USB 1") -> ("JoystickDevRef"=w28:T17)  [unwired: 10 in]
  n87 = call <vilib>:"WPI_JoystickRefNum Registry Set.vi"("refnum name"="Controller", "JoystickDevRef"=w29) -> ("JoystickDevRef"=w24:T17)  [unwired: 8 in, 1 out]
  n88 = call <vilib>:"WPI_JoystickRefNum Registry Set.vi"("refnum name"="Y Joystick", "JoystickDevRef"=w28) -> ("JoystickDevRef"=w25:T17)  [unwired: 8 in, 1 out]
  n89 = call <vilib>:"WPI_JoystickRefNum Registry Set.vi"("refnum name"="X Joystick", "JoystickDevRef"=w27) -> ("JoystickDevRef"=w26:T17)  [unwired: 8 in, 1 out]
  n90 = Bundle By Name(cluster="Teleop/Auto output cluster", "Gyro"=w63, "Right Drive Encoder"=w64, "Left Drive Encoder"=w65, "X Joystick"=w26, "Y Joystick"=w25, "Controller"=w24, "DriveMotors"=w66) -> (→"Teleop/Auto output cluster out":T16)
  "error out" <- "error in"
